vi "Fetch Messages.vi"(8 "error in (no error)":errorcluster, 9 "Remainder In":string, 11 "VISA resource name":refnum<visa-resource-name>) -> (0 "error out":errorcluster, 1 "Remainder Out":string, 2 "Complete Messages":string[](array[string]), 3 "VISA resource name out":refnum<visa-resource-name>)   [LabVIEW 2012, in "MicroStrain 3DM-GXx.lvlib"]
doc: "Read the input buffer and create an array of complete messages received."
uses:
  <instrlib>/MicroStrain 3DM-GXx/MicroStrain 3DM-GXx.lvlib
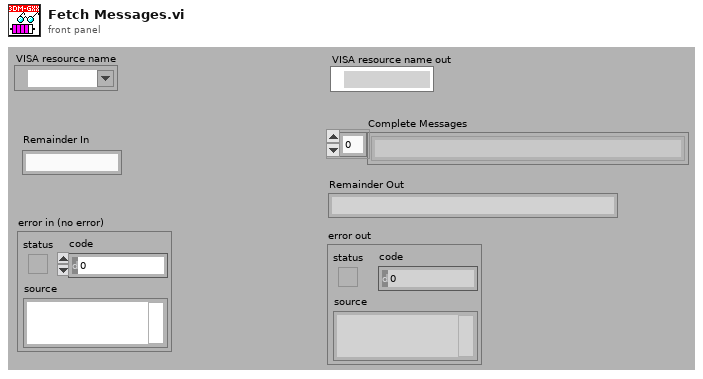
[diagram p1: front panel]
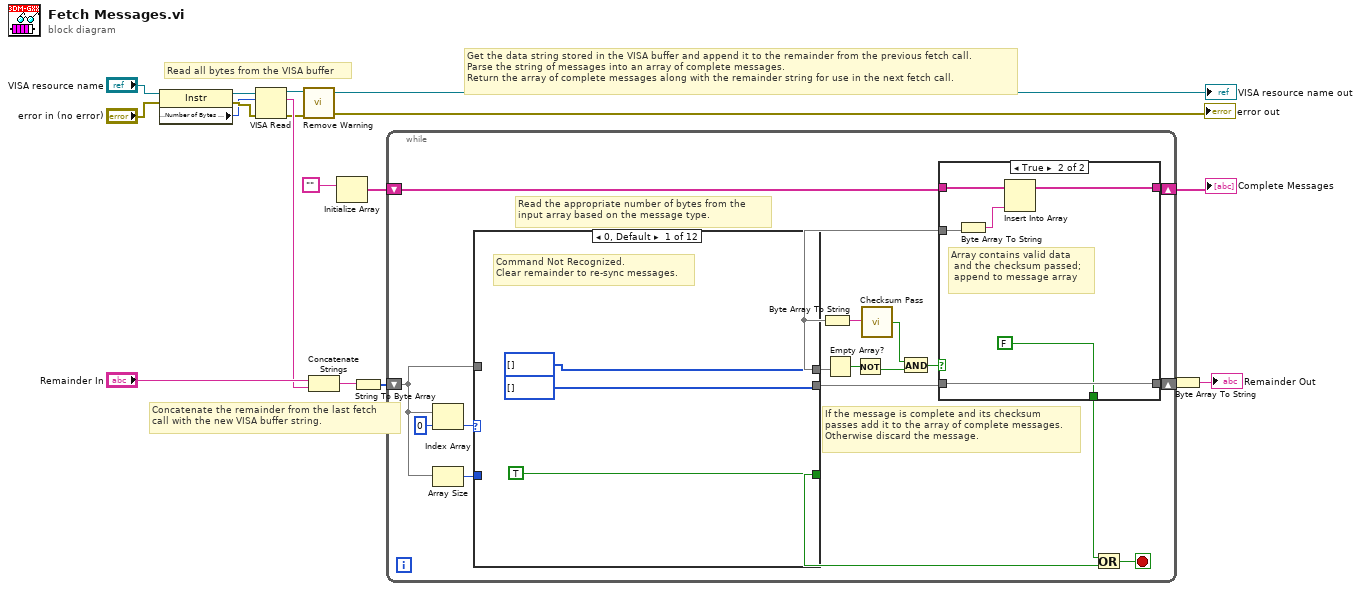
[diagram p0: block diagram]
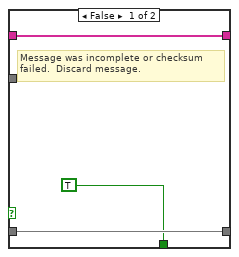
[diagram p2: hidden frame]
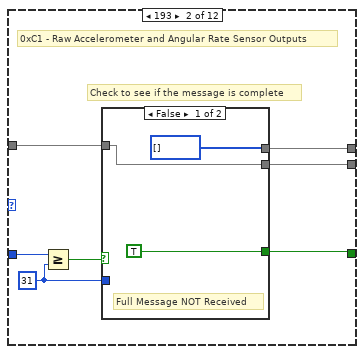
[diagram p3: hidden frame]
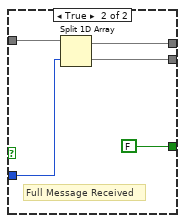
[diagram p4: hidden frame]
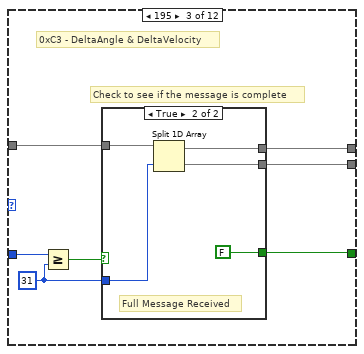
[diagram p5: hidden frame]
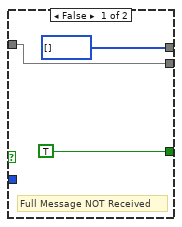
[diagram p6: hidden frame]
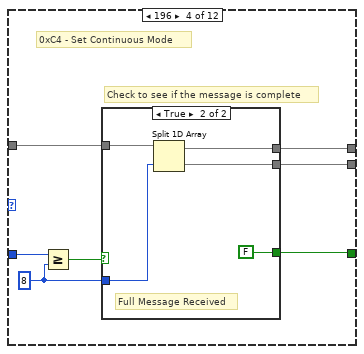
[diagram p7: hidden frame]
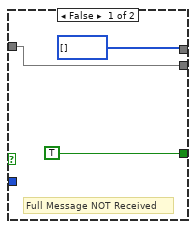
[diagram p8: hidden frame]
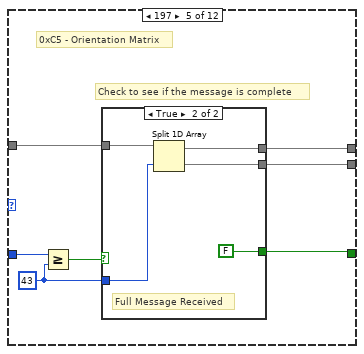
[diagram p9: hidden frame]
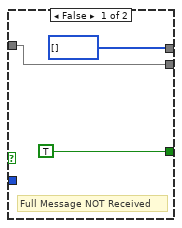
[diagram p10: hidden frame]
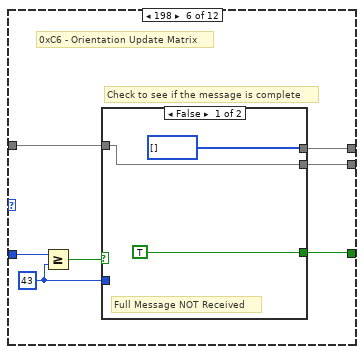
[diagram p11: hidden frame]
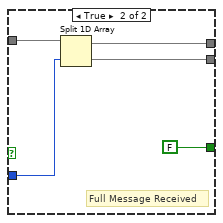
[diagram p12: hidden frame]
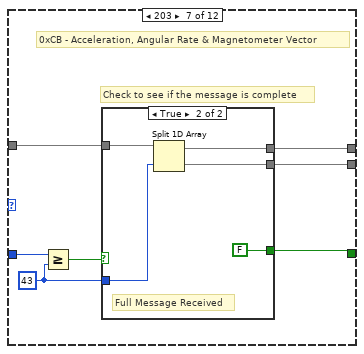
[diagram p13: hidden frame]
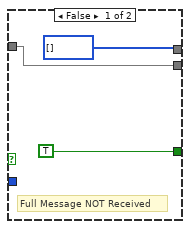
[diagram p14: hidden frame]
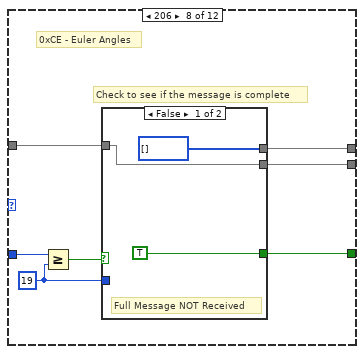
[diagram p15: hidden frame]
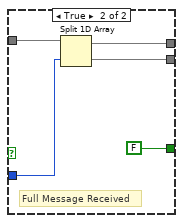
[diagram p16: hidden frame]
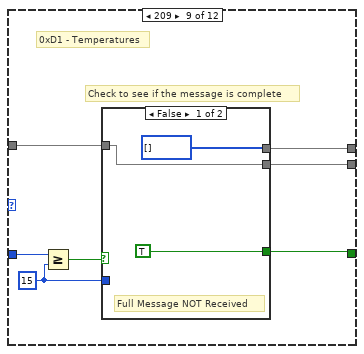
[diagram p17: hidden frame]
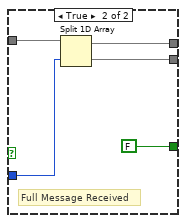
[diagram p18: hidden frame]
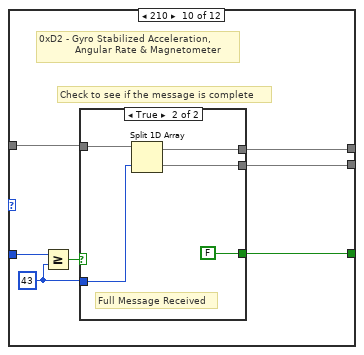
[diagram p19: hidden frame]
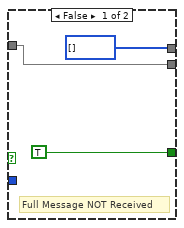
[diagram p20: hidden frame]
diagram:
  # "Get the data string stored in the VISA buffer and append it to the remainder from the previous fetch call. \nParse the string of messages into an array of complete messages.\nReturn the array of complete messages along with the remainder string for use in the next fetch call."
  # "Concatenate the remainder from the last fetch \ncall with the new VISA buffer string."
  # "Read all bytes from the VISA buffer"
  n1 = property class="Instr"(reference="VISA resource name", error in="error in (no error)") -> (reference out=w17:refnum<visa-resource-name>, error out=w16:errorcluster, "Serial Settings:Number of Bytes at Serial Port"=w5:u32)
  n2 = VISA Read(VISA resource name=w17, byte count=w5, error in (no error)=w16) -> (VISA resource name out=w4:refnum<visa-resource-name>, read buffer=w6:string, error out=w3:errorcluster)  [unwired: 1 out]
  n3 = call <instrlib>:"Remove Warning.vi"("error in (no error)"=w3, "VISA resource name"=w4) -> ("error out"=→"error out":errorcluster, "VISA resource name out"=→"VISA resource name out":refnum<visa-resource-name>)  [unwired: 2 in]
  n4 = Concatenate Strings("Remainder In", w6) -> (w13:string)
  n5 = Initialize Array("") -> (w11:string[])  [unwired: 1 in]
  n6 = String To Byte Array(string=w13) -> (unsigned byte array=w12:u8[])
  n7 = while {
    shift-right: [w30] -> w8
    shift-left: w12 -> [w34]
    shift-right: [w31] -> w9
    shift-left: w11 -> [w32]
    stop <- w21 stop-if-true
    # "If the message is complete and its checksum\npasses add it to the array of complete messages.\nOtherwise discard the message."
    # "Read the appropriate number of bytes from the \ninput array based on the message type."
    n8 = Index Array(array=w34, index=0) -> (element=w28:u8)
    n9 = Array Size(array=w34) -> (size(s)=w33:i32)
    n10 = case shown="0, Default" w28 {
      tunnel: w34 -> [_ w52 w67 w82 w97 w112 w127 w142 w157 w172 w187 w202]
      tunnel: w33 -> [_ w54 w69 w84 w99 w114 w129 w144 w159 w174 w189 w204]
      tunnel: [u8[] [] w50 w65 w80 w95 w110 w125 w140 w155 w170 w185 w200] -> w26
      tunnel: [u8[] [] ("unsigned byte array") w49 w64 w79 w94 w109 w124 w139 w154 w169 w184 w199] -> w29
      tunnel: [TRUE ("Stop") w48 w63 w78 w93 w108 w123 w138 w153 w168 w183 w198] -> w19
      frame 0, Default {
        # "Command Not Recognized. \nClear remainder to re-sync messages."
      }
      frame 193 {
        w51 = 31
        # "Check to see if the message is complete"
        # "0xC1 - Raw Accelerometer and Angular Rate Sensor Outputs"
        n11 = Greater Or Equal?(x=w54, y=w51) -> (x >= y?=w53:bool)
        n12 = case shown="False" w53 {
          tunnel: w52 -> [w57 w62]
          tunnel: w51 -> [_ w61]
          tunnel: [u8[] [] w60] -> w50
          tunnel: [w57 w59] -> w49
          tunnel: [TRUE ("stop") FALSE ("stop")] -> w48
          frame False {
            # "Full Message NOT Received"
          }
          frame True {
            # "Full Message Received"
            n13 = Split 1D Array(array=w62, index=w61) -> (first subarray=w60:u8[], second subarray=w59:u8[])
          }
        }
      }
      frame 195 {
        w66 = 31
        # "Check to see if the message is complete"
        # "0xC3 - DeltaAngle & DeltaVelocity"
        n14 = Greater Or Equal?(x=w69, y=w66) -> (x >= y?=w68:bool)
        n15 = case shown="True" w68 {
          tunnel: w67 -> [w72 w77]
          tunnel: w66 -> [_ w76]
          tunnel: [u8[] [] w75] -> w65
          tunnel: [w72 w74] -> w64
          tunnel: [TRUE ("stop") FALSE ("stop")] -> w63
          frame False {
            # "Full Message NOT Received"
          }
          frame True {
            # "Full Message Received"
            n16 = Split 1D Array(array=w77, index=w76) -> (first subarray=w75:u8[], second subarray=w74:u8[])
          }
        }
      }
      frame 196 {
        w81 = 8
        # "Check to see if the message is complete"
        # "0xC4 - Set Continuous Mode"
        n17 = Greater Or Equal?(x=w84, y=w81) -> (x >= y?=w83:bool)
        n18 = case shown="True" w83 {
          tunnel: w82 -> [w87 w92]
          tunnel: w81 -> [_ w91]
          tunnel: [u8[] [] w90] -> w80
          tunnel: [w87 w89] -> w79
          tunnel: [TRUE ("stop") FALSE ("stop")] -> w78
          frame False {
            # "Full Message NOT Received"
          }
          frame True {
            # "Full Message Received"
            n19 = Split 1D Array(array=w92, index=w91) -> (first subarray=w90:u8[], second subarray=w89:u8[])
          }
        }
      }
      frame 197 {
        w96 = 43
        # "Check to see if the message is complete"
        # "0xC5 - Orientation Matrix"
        n20 = Greater Or Equal?(x=w99, y=w96) -> (x >= y?=w98:bool)
        n21 = case shown="True" w98 {
          tunnel: w97 -> [w102 w107]
          tunnel: w96 -> [_ w106]
          tunnel: [u8[] [] w105] -> w95
          tunnel: [w102 w104] -> w94
          tunnel: [TRUE ("stop") FALSE ("stop")] -> w93
          frame False {
            # "Full Message NOT Received"
          }
          frame True {
            # "Full Message Received"
            n22 = Split 1D Array(array=w107, index=w106) -> (first subarray=w105:u8[], second subarray=w104:u8[])
          }
        }
      }
      frame 198 {
        w111 = 43
        # "Check to see if the message is complete"
        # "0xC6 - Orientation Update Matrix"
        n23 = Greater Or Equal?(x=w114, y=w111) -> (x >= y?=w113:bool)
        n24 = case shown="False" w113 {
          tunnel: w112 -> [w117 w122]
          tunnel: w111 -> [_ w121]
          tunnel: [u8[] [] w120] -> w110
          tunnel: [w117 w119] -> w109
          tunnel: [TRUE ("stop") FALSE ("stop")] -> w108
          frame False {
            # "Full Message NOT Received"
          }
          frame True {
            # "Full Message Received"
            n25 = Split 1D Array(array=w122, index=w121) -> (first subarray=w120:u8[], second subarray=w119:u8[])
          }
        }
      }
      frame 203 {
        w126 = 43
        # "Check to see if the message is complete"
        # "0xCB - Acceleration, Angular Rate & Magnetometer Vector"
        n26 = Greater Or Equal?(x=w129, y=w126) -> (x >= y?=w128:bool)
        n27 = case shown="True" w128 {
          tunnel: w127 -> [w132 w137]
          tunnel: w126 -> [_ w136]
          tunnel: [u8[] [] w135] -> w125
          tunnel: [w132 w134] -> w124
          tunnel: [TRUE ("stop") FALSE ("stop")] -> w123
          frame False {
            # "Full Message NOT Received"
          }
          frame True {
            # "Full Message Received"
            n28 = Split 1D Array(array=w137, index=w136) -> (first subarray=w135:u8[], second subarray=w134:u8[])
          }
        }
      }
      frame 206 {
        w141 = 19
        # "Check to see if the message is complete"
        # "0xCE - Euler Angles"
        n29 = Greater Or Equal?(x=w144, y=w141) -> (x >= y?=w143:bool)
        n30 = case shown="False" w143 {
          tunnel: w142 -> [w147 w152]
          tunnel: w141 -> [_ w151]
          tunnel: [u8[] [] w150] -> w140
          tunnel: [w147 w149] -> w139
          tunnel: [TRUE ("stop") FALSE ("stop")] -> w138
          frame False {
            # "Full Message NOT Received"
          }
          frame True {
            # "Full Message Received"
            n31 = Split 1D Array(array=w152, index=w151) -> (first subarray=w150:u8[], second subarray=w149:u8[])
          }
        }
      }
      frame 209 {
        w156 = 15
        # "Check to see if the message is complete"
        # "0xD1 - Temperatures"
        n32 = Greater Or Equal?(x=w159, y=w156) -> (x >= y?=w158:bool)
        n33 = case shown="False" w158 {
          tunnel: w157 -> [w162 w167]
          tunnel: w156 -> [_ w166]
          tunnel: [u8[] [] w165] -> w155
          tunnel: [w162 w164] -> w154
          tunnel: [TRUE ("stop") FALSE ("stop")] -> w153
          frame False {
            # "Full Message NOT Received"
          }
          frame True {
            # "Full Message Received"
            n34 = Split 1D Array(array=w167, index=w166) -> (first subarray=w165:u8[], second subarray=w164:u8[])
          }
        }
      }
      frame 210 {
        w171 = 43
        # "Check to see if the message is complete"
        # "0xD2 - Gyro Stabilized Acceleration,\n            Angular Rate & Magnetometer"
        n35 = Greater Or Equal?(x=w174, y=w171) -> (x >= y?=w173:bool)
        n36 = case shown="True" w173 {
          tunnel: w172 -> [w177 w182]
          tunnel: w171 -> [_ w181]
          tunnel: [u8[] [] w180] -> w170
          tunnel: [w177 w179] -> w169
          tunnel: [TRUE ("stop") FALSE ("stop")] -> w168
          frame False {
            # "Full Message NOT Received"
          }
          frame True {
            # "Full Message Received"
            n37 = Split 1D Array(array=w182, index=w181) -> (first subarray=w180:u8[], second subarray=w179:u8[])
          }
        }
      }
      frame 228 {
        w186 = 5
        # "Check to see if the message is complete"
        # "0xE4 - Write Word To eeprom"
        n38 = Greater Or Equal?(x=w189, y=w186) -> (x >= y?=w188:bool)
        n39 = case shown="True" w188 {
          tunnel: w187 -> [w192 w197]
          tunnel: w186 -> [_ w196]
          tunnel: [u8[] [] w195] -> w185
          tunnel: [w192 w194] -> w184
          tunnel: [TRUE ("stop") FALSE ("stop")] -> w183
          frame False {
            # "Full Message NOT Received"
          }
          frame True {
            # "Full Message Received"
            n40 = Split 1D Array(array=w197, index=w196) -> (first subarray=w195:u8[], second subarray=w194:u8[])
          }
        }
      }
      frame 229 {
        w201 = 5
        # "Check to see if the message is complete"
        # "0xE5 - Read Word from EEPROM"
        n41 = Greater Or Equal?(x=w204, y=w201) -> (x >= y?=w203:bool)
        n42 = case shown="False" w203 {
          tunnel: w202 -> [w207 w212]
          tunnel: w201 -> [_ w211]
          tunnel: [u8[] [] w210] -> w200
          tunnel: [w207 w209] -> w199
          tunnel: [TRUE ("stop") FALSE ("stop")] -> w198
          frame False {
            # "Full Message NOT Received"
          }
          frame True {
            # "Full Message Received"
            n43 = Split 1D Array(array=w212, index=w211) -> (first subarray=w210:u8[], second subarray=w209:u8[])
          }
        }
      }
    }
    n44 = Byte Array To String(unsigned byte array=w26) -> (string=w25:string)
    n45 = Empty Array?(array=w26) -> (empty?=w27:bool)
    n46 = Not(x=w27) -> (.not. x?=w22:bool)
    n47 = call <instrlib>:"Checksum Pass.vi"("Message In"=w25) -> ("Checksum Pass"=w23:bool)  [unwired: 4 in]
    n48 = And(x=w23, y=w22) -> (x .and. y?=w24:bool)
    n49 = case shown="True" w24 {
      tunnel: w32 -> [w38 w43]
      tunnel: w26 -> [_ w42]
      tunnel: [w38 w41] -> w31
      tunnel: [w37 w40] -> w30
      tunnel: w29 -> [w37 w40]
      tunnel: [TRUE ("stop") FALSE ("stop")] -> w20
      frame False {
        # "Message was incomplete or checksum\nfailed.  Discard message."
      }
      frame True {
        # "Array contains valid data\n and the checksum passed;\n append to message array"
        n50 = Byte Array To String(unsigned byte array=w42) -> (string=w44:string)
        n51 = Insert Into Array(array=w43, new element=w44) -> (w41:string[])  [unwired: 1 in]
      }
    }
    n52 = Or(x=w20, y=w19) -> (x .or. y?=w21:bool)
  }
  "Complete Messages" <- w9
  n53 = Byte Array To String(unsigned byte array=w8) -> (string=→"Remainder Out":string)
